vi "DynamicLoadLRvi.vi"() -> ()   [LabVIEW 2020]
panel:
  out "控件值:获取全部":cluster{"Name":string, "Variant Data":variant}[](array[cluster])
  in  "校验长度":u8
  in  "校验数据":u8[](array[numeric])
  in  "校验算法名称":string="Anti_Add"
  in  "LibName\\viName":string="LibFromLR"
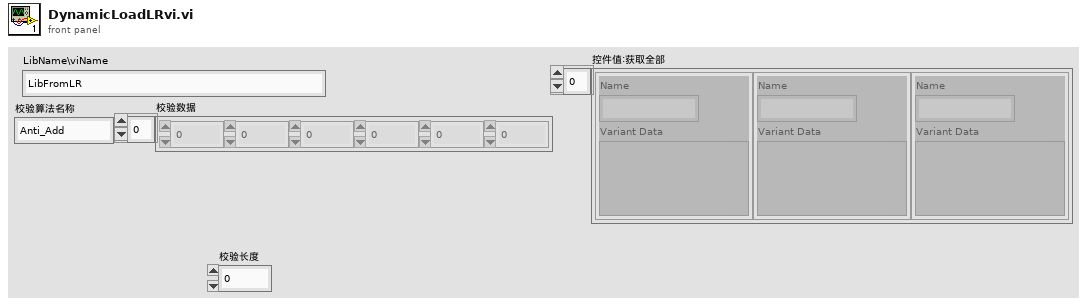
[diagram p1: front panel]
types:
  T1 = enum32{"invalid app kind", "Development System", "Run Time System", "Student Edition", "Embedded LabVIEW", "Evaluation", "Custom"}
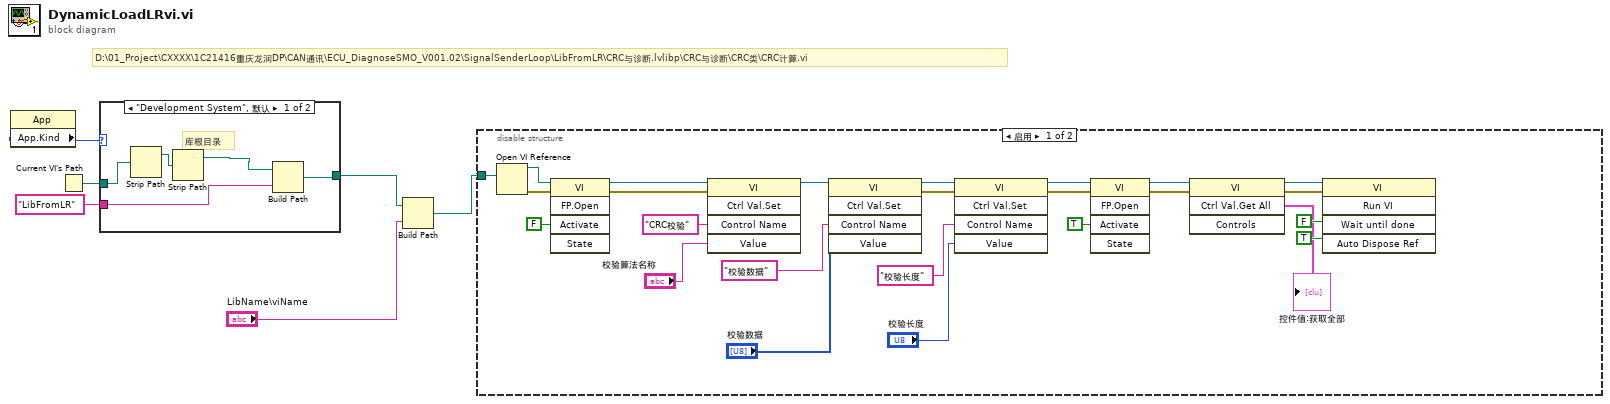
[diagram p0: block diagram]
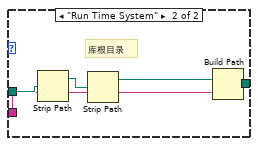
[diagram p3: hidden frame]
diagram:
  # "D:\\01_Project\\CXXXX\\1C21416重庆龙润DP\\CAN通讯\\ECU_DiagnoseSMO_V001.02\\SignalSenderLoop\\LibFromLR\\CRC与诊断.lvlibp\\CRC与诊断\\CRC类\\CRC计算.vi"
  n1 = property class="App"() -> ("App.Kind"=w4:T1)  [unwired: 2 in, 2 out]
  n2 = Current VI's Path() -> (path=w5:path)
  n3 = case shown="\"Development System\", 默认" w4 {
    tunnel: w5 -> [w11 w16]
    tunnel: [w8 w12] -> w3
    tunnel: "LibFromLR" ("ConfigFlieFolderName") -> [w7 w13]
    frame "Development System", Default {
      # "库根目录"
      n4 = Strip Path(path=w11) -> (stripped path=w10:path)  [unwired: 1 out]
      n5 = Strip Path(path=w10) -> (stripped path=w9:path)  [unwired: 1 out]
      n6 = Build Path(base path=w9, name or relative path=w7) -> (appended path=w8:path)
    }
    frame "Run Time System" {
      # "库根目录"
      n7 = Strip Path(path=w16) -> (stripped path=w15:path)  [unwired: 1 out]
      n8 = Strip Path(path=w15) -> (stripped path=w14:path)  [unwired: 1 out]
      n9 = Build Path(base path=w14, name or relative path=w13) -> (appended path=w12:path)
    }
  }
  n10 = Build Path(base path=w3, name or relative path="LibName\\viName") -> (appended path=w1:path)
  n11 = disable-structure shown="启用" {
    disable-tunnel: w1 -> [w29 _]
    frame Enabled {
      n12 = Open VI Reference(vi path=w29) -> (vi reference=w40:refnum<vi>, error out=w41:errorcluster)  [unwired: 5 in]
      n13 = invoke class="VI" method="FP.Open"(reference=w40, error in=w41, "Activate"=FALSE ("激活？")) -> (reference out=w36:refnum<vi>, error out=w39:errorcluster)  [unwired: 2 in, 3 out]
      n14 = invoke class="VI" method="Ctrl Val.Set"(reference=w36, error in=w39, "Control Name"="CRC校验" ("控件名"), "Value"="校验算法名称") -> (reference out=w27:refnum<vi>)  [unwired: 1 in, 4 out]
      n15 = invoke class="VI" method="Ctrl Val.Set"(reference=w27, "Control Name"="校验数据" ("控件名"), "Value"="校验数据") -> (reference out=w26:refnum<vi>, error out=w25:errorcluster)  [unwired: 2 in, 3 out]
      n16 = invoke class="VI" method="Ctrl Val.Set"(reference=w26, error in=w25, "Control Name"="校验长度" ("控件名"), "Value"="校验长度") -> (reference out=w22:refnum<vi>, error out=w21:errorcluster)  [unwired: 1 in, 3 out]
      n17 = invoke class="VI" method="FP.Open"(reference=w22, error in=w21, "Activate"=TRUE ("激活？")) -> (reference out=w35:refnum<vi>, error out=w34:errorcluster)  [unwired: 2 in, 3 out]
      n18 = invoke class="VI" method="Ctrl Val.Get All"(reference=w35, error in=w34) -> (reference out=w33:refnum<vi>, error out=w32:errorcluster, "Get All Control Values Variant"=→"控件值:获取全部":cluster{"Name":string, "Variant Data":variant}[])  [unwired: 2 in, 1 out]
      n19 = invoke class="VI" method="Run VI"(reference=w33, error in=w32, "Wait until done"=FALSE ("Wait Until Done"), "Auto Dispose Ref"=TRUE ("Auto Dispose Reference")) -> ()  [unwired: 1 in, 5 out]
    }
    frame Disabled {
    }
  }
